vi "mod_Set Error Source.vi"(3 "initial error in (no error)":errorcluster, 5 "final error in (no error)":errorcluster) -> (2 "error out":errorcluster)   [LabVIEW 2020, in "niAMT.lvlib"]
doc: "This VI compares the error in (to the calling VI) with the error out (of the calling VI). If they are different (the calling VI generated an error) this VI sets the error source to be the call chain of the calling VI."
uses:
  <vilib>/addons/Modulation/niAMT.lvlib
panel:
  # "This VI compares the error in (to the calling VI) with the error out (of the calling VI).  If they are different (the calling VI generated an error) this VI sets the error source to be the call chain of the calling VI."
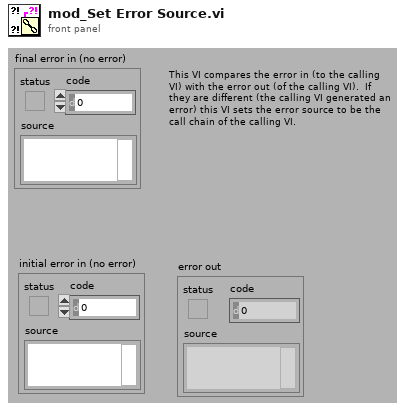
[diagram p1: front panel]
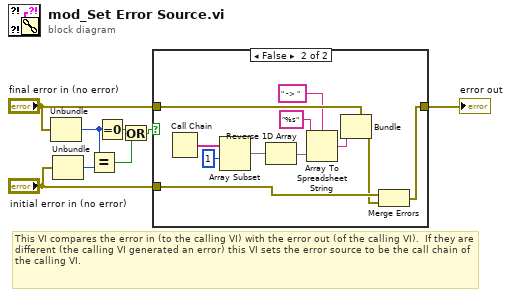
[diagram p0: block diagram]
diagram:
  # "This VI compares the error in (to the calling VI) with the error out (of the calling VI).  If they are different (the calling VI generated an error) this VI sets the error source to be the call chain of the calling VI."
  n1 = Unbundle("final error in (no error)") -> ("code"=w2:i32)  [unwired: 2 out]
  n2 = Unbundle("initial error in (no error)") -> ("code"=w3:i32)  [unwired: 2 out]
  n3 = Equal?(x=w2, y=w3) -> (x = y?=w1:bool)
  n4 = Equal To 0?(x=w2) -> (x = 0?=w7:bool)
  n5 = Or(x=w7, y=w1) -> (x .or. y?=w5:bool)
  n6 = case shown="False" w5 {
    tunnel: [w9 w10] -> w8
    tunnel: "final error in (no error)" -> [_ w18]
    tunnel: "initial error in (no error)" -> [w9 w12]
    frame True {
    }
    frame False {
      n7 = Call Chain() -> (call chain=w20:string[])
      n8 = Array Subset(array=w20, index=1) -> (w14:string[])  [unwired: 1 in]
      n9 = Reverse 1D Array(array=w14) -> (reversed array=w13:string[])
      n10 = Array To Spreadsheet String(delimiter (Tab)=" -> ", array=w13, 3:"%s" ("format string")) -> (spreadsheet string=w17:string)
      n11 = Bundle(cluster=w18, "source"=w17) -> (w11:errorcluster)  [unwired: 2 out]
      n12 = Merge Errors(w12, w11) -> (w10:errorcluster)
    }
  }
  "error out" <- w8
